vi "GetAncestorClass.vi"(1 "LabVIEWClass":refnum<vi>, 5 "error in (no error)":errorcluster) -> (15 "Ancestor":refnum<vi>, 19 "error out":errorcluster)   [LabVIEW 2017, in "G#IDE.lvlib" / "LibraryLib.lvlib"]
uses:
  <resource>/Framework/Providers/AddQ/G#IDE/support/LibraryLib/LibraryLib.lvlib
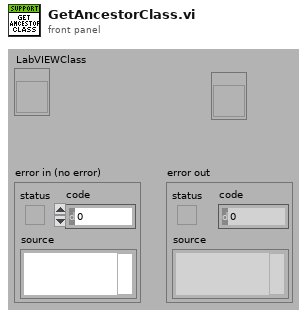
[diagram p1: front panel]
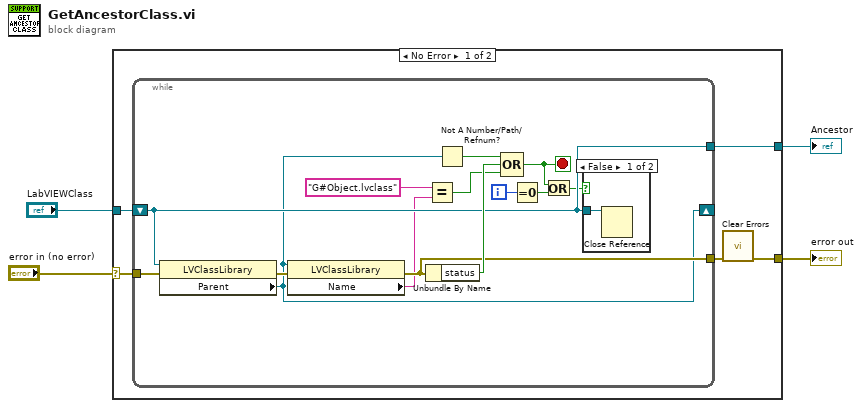
[diagram p0: block diagram]
diagram:
  n1 = case shown="No Error" "error in (no error)" {
    selector: "error in (no error)" -> [w7 w25]
    tunnel: [w6 w25] -> w4
    tunnel: "LabVIEWClass" -> [w9 _]
    tunnel: [w8 _] -> w1
    frame No Error {
      n2 = while {
        shift-right: [w10] -> _
        shift-left: w9 -> [w20]
        tunnel: w7 -> [w21]
        tunnel: [w12] -> w5
        tunnel: [w20] -> w8
        i -> [w17]
        stop <- w19 stop-if-true
        n3 = property class="LVClassLibrary"(reference=w20, error in=w21) -> (error out=w13:errorcluster, "Parent"=w10:refnum<vi>)  [unwired: 1 out]
        n4 = property class="LVClassLibrary"(reference=w10, error in=w13) -> (error out=w12:errorcluster, "Name"=w11:string)  [unwired: 1 out]
        n5 = Unbundle By Name(w12) -> ("status"=w22:bool)
        n6 = Equal?(x="G#Object.lvclass" ("y"), y=w11) -> (x = y?=w14:bool)
        n7 = Not A Number/Path/Refnum?(number/path/refnum=w10) -> (NaN/Path/Refnum?=w23:bool)
        n8 = Compound Arithmetic op=OR(w23, w22, w14) -> (w19:bool)
        n9 = Equal To 0?(x=w17) -> (x = 0?=w16:bool)
        n10 = Or(x=w19, y=w16) -> (x .or. y?=w18:bool)
        n11 = case shown="False" w18 {
          tunnel: w20 -> [w24 _]
          frame False {
            n12 = Close Reference(reference=w24) -> ()  [unwired: 1 in, 1 out]
          }
          frame True {
          }
        }
      }
      n13 = call <vilib>:"Clear Errors.vi"("error in (no error)"=w5) -> ("error out"=w6:errorcluster)  [unwired: 5 in, 1 out]
    }
    frame Error {
    }
  }
  "error out" <- w4
  "Ancestor" <- w1
